vi "TDK电流加载.vi"(8 "error in (no error)":errorcluster, 9 "时间(s)":dbl=1.0 caption="延迟时间(s)", 10 "电流":dbl format="%.4f", 11 "VISA resource name":refnum<visa-resource-name>) -> (0 "error out":errorcluster caption="错误输出", 3 "VISA resource name out":refnum<visa-resource-name>)   [LabVIEW 2021]
uses:
  <instrlib>/TDK-Lambda G Series/TDK-Lambda G Series.lvlib
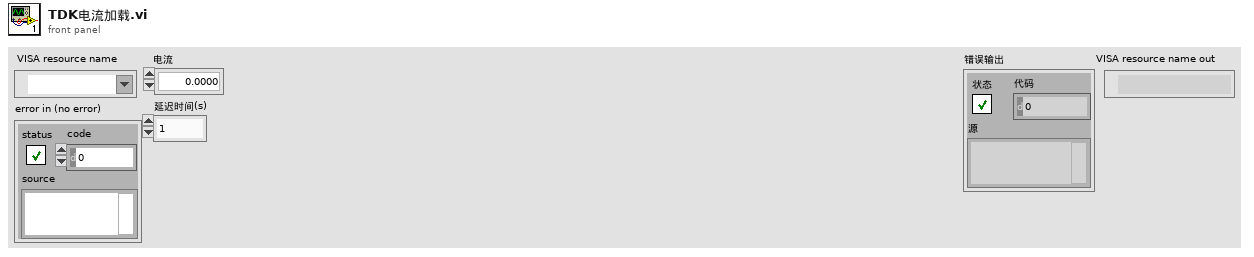
[diagram p1: front panel]
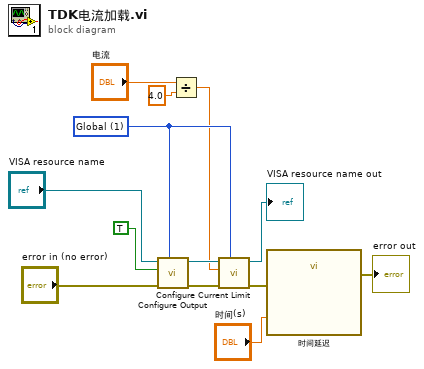
[diagram p0: block diagram]
diagram:
  w4 = u16 1 items=["Single", "Global"] ("Globalize (0: Single)")
  n1 = call <instrlib>:"Configure Output.vi"("Globalize (0: Single)"=w4, "error in (no error)"="error in (no error)", "Enable Output (False)"=TRUE, "VISA resource name"="VISA resource name") -> ("error out"=w10:errorcluster, "VISA resource name out"=w11:refnum<visa-resource-name>)  [unwired: 6 in]
  n2 = Divide(x="电流", y=4.0) -> (x/y=w1:dbl)
  n3 = call <instrlib>:"Configure Current Limit.vi"("Globalize (0: Single)"=w4, "error in (no error)"=w10, "Current Limit (0A)"=w1, "VISA resource name"=w11) -> ("error out"=w9:errorcluster, "VISA resource name out"=→"VISA resource name out":refnum<visa-resource-name>)  [unwired: 6 in]
  n4 = call "时间延迟"("error in (no error)"=w9, "Delay Time (s)"="时间(s)") -> ("error out"=→"error out":errorcluster)  [unwired: 9 in]
